vi "visual_test.vi"() -> ()   [LabVIEW 2017]
doc: "Demonstrates how to programmatically move Front Panel elements with drag and drop mouse gestures"
uses:
  <vilib>/Utility/miscctls.llb/LVPoint32TypeDef.ctl
panel:
  in  "New Coords":T1
  in  "stop 3":bool
  in  "stop 2":bool
  in  "reference out":refnum<vi>
  out "Cluster":T2
  in  "stop":bool
  out "Movable Gauge":dbl
  # "Overview: Demonstrates how to programmatically move Front Panel elements with drag and drop mouse gestures\nRequirements: LabVIEW 2012 Base Development System (or compatible)\nInstructions: \n1. Run the VI\n2. Click on the Movable Gauge and release the mouse button where you want to move the Gauge to"
types:
  T1 = typedef "LVPoint32TypeDef.ctl" = cluster{"Horizontal":i32, "Vertical":i32}
  T2 = cluster{"TC 1":bool, "TC 2":bool, "TC 3":bool, "TC 4":bool, "TC 5":bool, "new picture":picture}
  T3 = typedef "LVPositionTypeDef.ctl" = cluster{"Left":i32, "Top":i32}
  T4 = typedef "imagedata.ctl" = cluster{"image type":i32, "image depth":i32, "image":u8[], "mask":u8[], "colors":u32[], "Rectangle":cluster{"left":i16, "top":i16, "right":i16, "bottom":i16}}
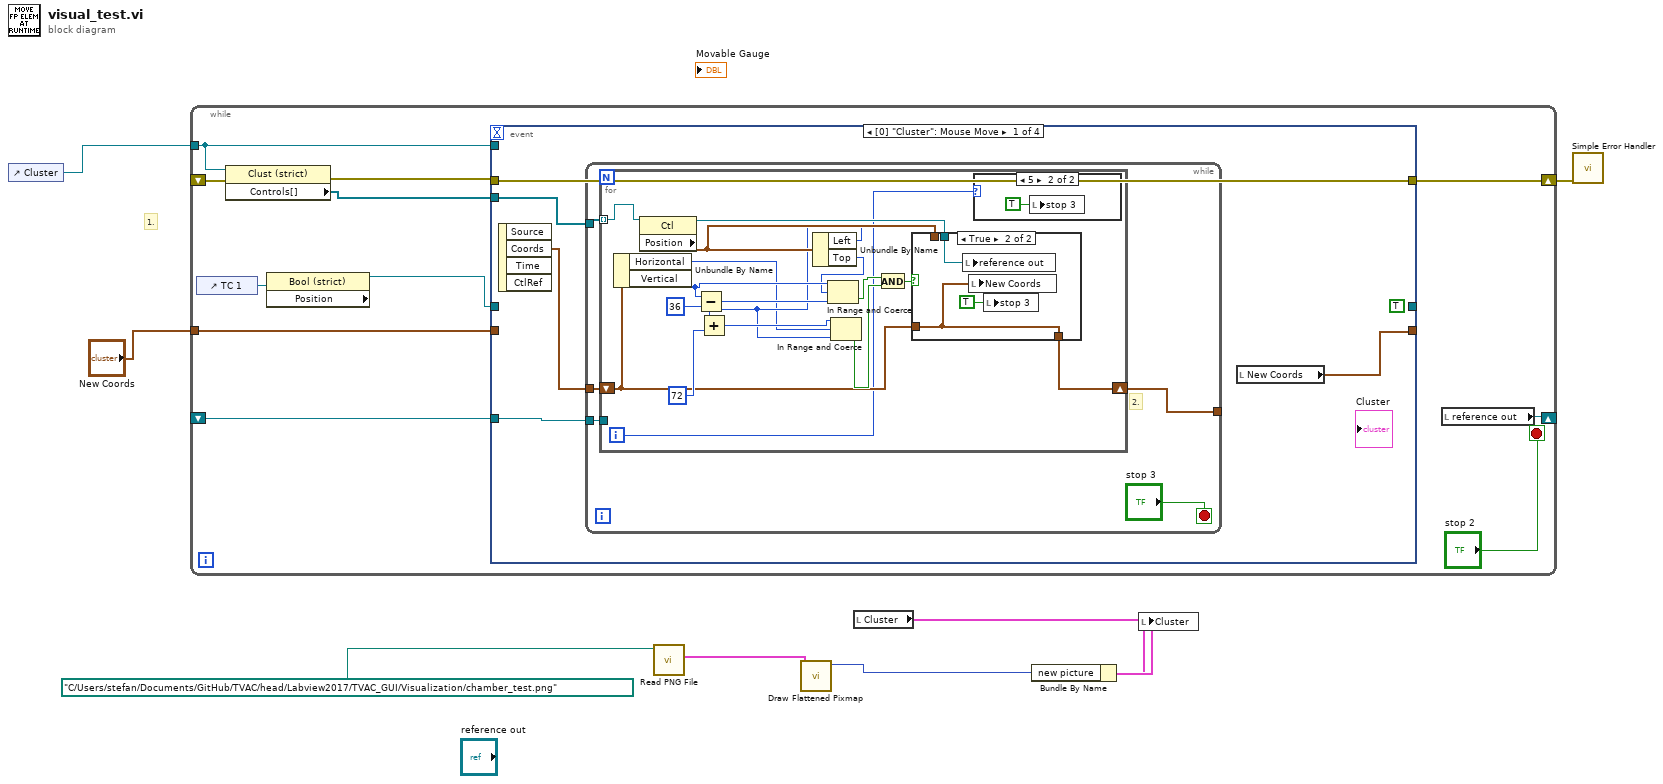
[diagram p0: block diagram]
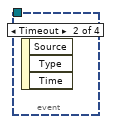
[diagram p4: hidden frame]
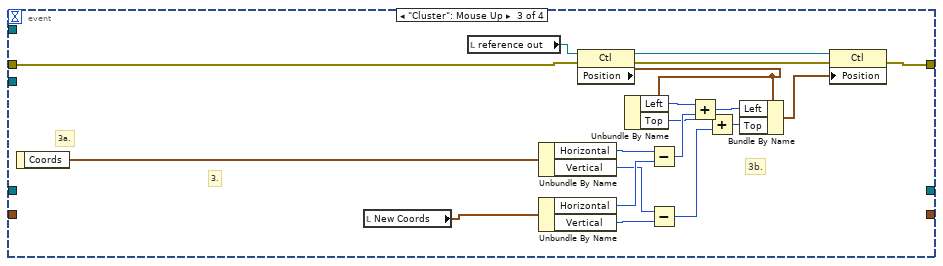
[diagram p5: hidden frame]
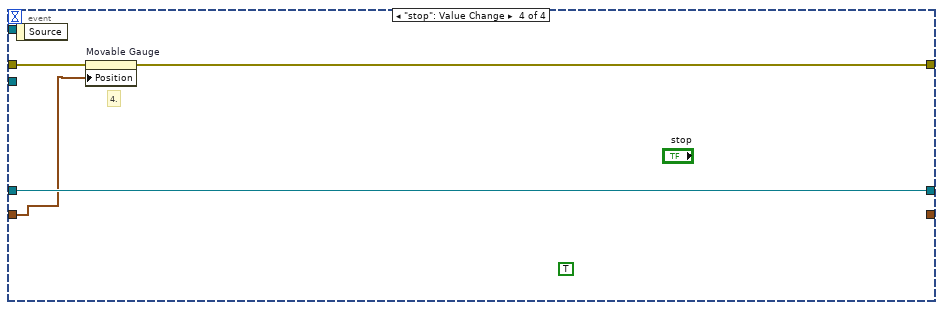
[diagram p6: hidden frame]
diagram:
  # "1."
  n1 = control-ref of="Cluster"() -> (w5:refnum<vi>)
  n2 = while {
    shift-right: [w19] -> w8
    shift-left: _ -> [w11]
    tunnel: w5 -> [w13]
    shift-right: [w17] -> _
    shift-left: _ -> [w18]
    tunnel: "New Coords" -> [w9]
    stop <- "stop 2" stop-if-true
    n3 = control-ref of="TC 1"() -> (w15:refnum<vi>)
    n4 = property on="Property Node" class="Clust (strict)"(reference=w13, error in=w11) -> (error out=w10:errorcluster, "Controls[]"=w12:refnum<vi>[])  [unwired: 1 out]
    n5 = property class="Bool (strict)" props=["Position"](reference=w15) -> (reference out=w14:refnum<vi>)  [unwired: 1 in, 2 out]
    n6 = event shown="[0] \"Cluster\": Mouse Move" {
      selector: _ -> [_ _ _ _]
      dyn-events: _ -> [_ _ _ _]
      timeout: _ -> [_ _ _ _]
      tunnel: [w20 _ _ _] -> _
      tunnel: [_ _ _ w74] -> _
      tunnel: w14 -> [_ _ _ w74]
      tunnel: w9 -> [_ _ _ w71]
      tunnel: [w24 _ w69 w72] -> w19
      tunnel: w10 -> [w24 _ w68 w73]
      tunnel: w13 -> [_ _ _ _]
      tunnel: w12 -> [w21 _ _ _]
      tunnel: w18 -> [w22 _ _ _]
      event "Cluster": Mouse Move {
        (unwired) TRUE
        n7 = event-data() -> ("Coords"=w23:T1)  [unwired: 4 out]
        n8 = while {
          tunnel: w23 -> [w29]
          tunnel: [w28] -> _
          tunnel: w22 -> [w27]
          tunnel: w21 -> [w26]
          stop <- "stop 3" stop-if-true
          # "2."
          n9 = for {
            shift-right: [w30] -> w28
            shift-left: w29 -> [w36]
            tunnel: w27 -> [_]
            tunnel: w26 -> [w34] mode=indexing
            i -> [w33]
            n10 = Unbundle By Name(w36) -> ("Horizontal"=w31:i32, "Vertical"=w44:i32)
            n11 = property class="Ctl"(reference=w34) -> (reference out=w35:refnum<vi>, "Position"=w37:T3)  [unwired: 1 in, 1 out]
            n12 = Subtract(x=w44, y=36) -> (x-y=w45:i32)
            n13 = Unbundle By Name(w37) -> ("Left"=w32:i32, "Top"=w43:i32)
            n14 = Add(x=w32, y=72) -> (x+y=w41:i32)
            n15 = In Range and Coerce(upper limit=w44, x=w43, lower limit=w45) -> (In Range?=w38:bool)  [unwired: 1 out]
            n16 = In Range and Coerce(upper limit=w41, x=w31, lower limit=w32) -> (In Range?=w39:bool)  [unwired: 1 out]
            n17 = And(x=w38, y=w39) -> (x .and. y?=w40:bool)
            n18 = case shown="True" w40 {
              tunnel: w37 -> [_ _]
              tunnel: [w48 w49] -> w30
              tunnel: w36 -> [w48 w49]
              tunnel: w35 -> [_ w51]
              frame False {
              }
              frame True {
                n19 = local write "reference out"(w51) -> ()
                n20 = local write "New Coords"(w49) -> ()
                n21 = local write "stop 3"(TRUE ("stop 3")) -> ()
              }
            }
            n22 = case shown="5" w33 {
              frame 0, Default {
              }
              frame 5 {
                n23 = local write "stop 3"(TRUE ("stop 3")) -> ()
              }
            }
          }
        }
        n24 = local read "New Coords"() -> (w20:T1)
      }
      event Timeout {
        n25 = event-data() -> ()  [unwired: 4 out]
      }
      event "Cluster": Mouse Up {
        # "3b."
        # "3a."
        # "3."
        n26 = event-data() -> ("Coords"=w70:T1)  [unwired: 1 out]
        n27 = local read "New Coords"() -> (w53:T1)
        n28 = local read "reference out"() -> (w52:refnum<vi>)
        n29 = Unbundle By Name(w70) -> ("Horizontal"=w67:i32, "Vertical"=w65:i32)
        n30 = Unbundle By Name(w53) -> ("Horizontal"=w66:i32, "Vertical"=w64:i32)
        n31 = property class="Ctl"(reference=w52, error in=w68) -> (reference out=w56:refnum<vi>, error out=w55:errorcluster, "Position"=w54:T3)
        n32 = Unbundle By Name(w54) -> ("Left"=w62:i32, "Top"=w61:i32)
        n33 = Subtract(x=w67, y=w66) -> (x-y=w63:i32)
        n34 = Subtract(x=w65, y=w64) -> (x-y=w60:i32)
        n35 = Add(x=w62, y=w63) -> (x+y=w58:i32)
        n36 = Add(x=w61, y=w60) -> (x+y=w59:i32)
        n37 = Bundle By Name(cluster=w54, "Left"=w58, "Top"=w59) -> (w57:T3)
        n38 = property on="Property Node" class="Ctl"(reference=w56, error in=w55, "Position"=w57) -> (error out=w69:errorcluster)  [unwired: 1 out]
      }
      event "stop": Value Change {
        (unwired) TRUE
        # "4."
        n39 = event-data() -> ()  [unwired: 2 out]
        n40 = property on="Movable Gauge" class="DigNum (strict)"(error in=w73, "Position"=w71) -> (error out=w72:errorcluster)  [unwired: 1 in, 1 out]
      }
    }
    n41 = local read "reference out"() -> (w17:refnum<vi>)
  }
  n42 = call <vilib>:"Read PNG File.vi"("path to PNG file"=path "C:/Users/stefan/Documents/GitHub/TVAC/head/Labview2017/TVAC_GUI/Visualization/chamber_test.png") -> ("image data"=w6:T4)  [unwired: 8 in, 2 out]
  n43 = call <vilib>:"Draw Flattened Pixmap.vi"("image data"=w6) -> ("new picture"=w2:picture)  [unwired: 8 in]
  n44 = local read "Cluster"() -> (w3:T2)
  n45 = Bundle By Name(cluster=w3, "new picture"=w2) -> (w4:T2)
  n46 = local write "Cluster"(w4) -> ()
  n47 = call <vilib>:"Simple Error Handler.vi"("error in (no error)"=w8) -> ()  [unwired: 4 in, 5 out]
